vi "GetParam.vi"(8 "error in (no error)":errorcluster caption="entrée d'erreur (pas d'erreur)", 11 "RBFSampler.lvclass":refnum<class "RBFSampler.lvclass">) -> (0 "error out":errorcluster caption="sortie d'erreur", 2 "RBFSampler":T1={"gamma"=1.0, "n_components"=100, "random_state"=-1} {"random_state" min=-1}, 3 "RBFSampler.lvclass":refnum<class "RBFSampler.lvclass">)   [LabVIEW 2020, in "RBFSampler.lvclass"]
doc: "Get Parameters"
uses:
  RBFSampler.lvclass
  RBFSampler.lvclass/RBFSampler.ctl
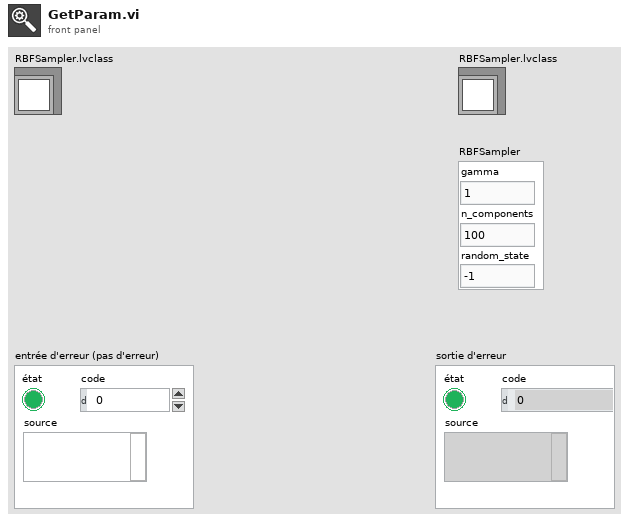
[diagram p1: front panel]
types:
  T1 = cluster{"gamma":dbl, "n_components":i32, "random_state":i32}
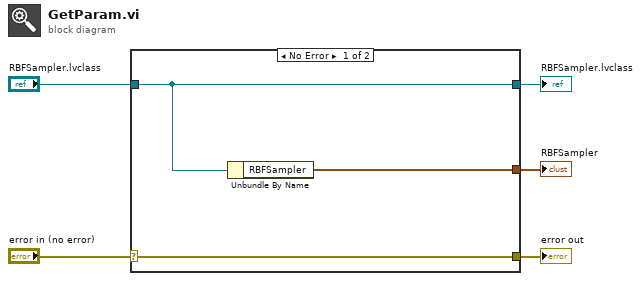
[diagram p0: block diagram]
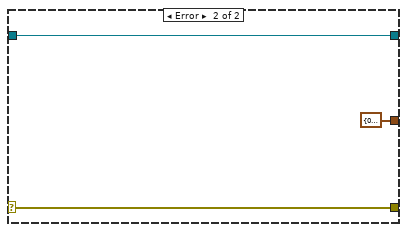
[diagram p2: hidden frame]
diagram:
  n1 = case shown="No Error" "error in (no error)" {
    selector: "error in (no error)" -> [w8 w10]
    tunnel: [w8 w10] -> w4
    tunnel: [w7 w11] -> w2
    tunnel: "RBFSampler.lvclass" -> [w7 w11]
    tunnel: [w6 T1 {"gamma"=0.0, "n_components"=0, "random_state"=0} ("RBFSampler")] -> w1
    frame No Error {
      n2 = Unbundle By Name(w7) -> ("RBFSampler"=w6:T1)
    }
    frame Error {
    }
  }
  "error out" <- w4
  "RBFSampler.lvclass" <- w2
  "RBFSampler" <- w1
